vi "stage 2.vi"() -> (0 "pass":bool=TRUE, 1 "Boolean 5":bool, 2 "Boolean 7":bool, 3 "Boolean 8":bool)   [LabVIEW 2014]
uses:
  <vilib>/Utility/miscctls.llb/LVPositionTypeDef.ctl
panel:
  in  "Position 2":T1={"Left"=264, "Top"=264}
  in  "hh":dbl format="%0#2_6g"
  in  ":":dbl format="%0#2_6g"
  in  "ss":dbl format="%0#2_6g"
  out "star 1":bool
  out "star 2":bool
  out "star 3":bool
  out "Boolean 3":bool
  out "Boolean":bool
  out "Boolean 2":bool
  out "Boolean 4":bool
  out "result":bool
  in  "Boolean 6":bool
  in  "Position":T1
  in  "character":bool
  in  "Map Array":dbl[][](array[numeric])=array120x120[14400 elements]
  in  "OK Button 44":bool
  in  "OK Button 43":bool
  in  "OK Button 42":bool
  in  "OK Button 41":bool
  in  "OK Button 40":bool
  in  "OK Button 39":bool
  in  "stop 2":bool
  in  "OK Button 38":bool
  in  "OK Button 37":bool
  in  "OK Button 36":bool
  in  "OK Button 35":bool
  in  "OK Button 34":bool
  in  "OK Button 33":bool
  in  "OK Button 32":bool
  in  "OK Button 29":bool
  in  "OK Button 31":bool
  in  "OK Button 28":bool
  in  "OK Button 27":bool
  in  "OK Button 30":bool
  in  "OK Button 26":bool
  in  "OK Button 25":bool
  in  "OK Button 24":bool
  in  "OK Button 23":bool
  in  "stop":bool
  in  "OK Button 22":bool
  in  "OK Button 21":bool
  in  "OK Button 20":bool
  in  "OK Button 19":bool
  in  "OK Button 18":bool
  in  "OK Button 17":bool
  in  "OK Button 16":bool
  in  "OK Button 15":bool
  in  "OK Button 14":bool
  in  "OK Button 13":bool
  in  "OK Button 12":bool
  in  "OK Button 11":bool
  in  "OK Button 10":bool
  in  "OK Button 9":bool
  in  "OK Button 8":bool
  in  "OK Button 7":bool
  in  "OK Button 6":bool
  in  "OK Button 5":bool
  in  "OK Button 4":bool
  in  "OK Button 3":bool
  in  "OK Button":bool
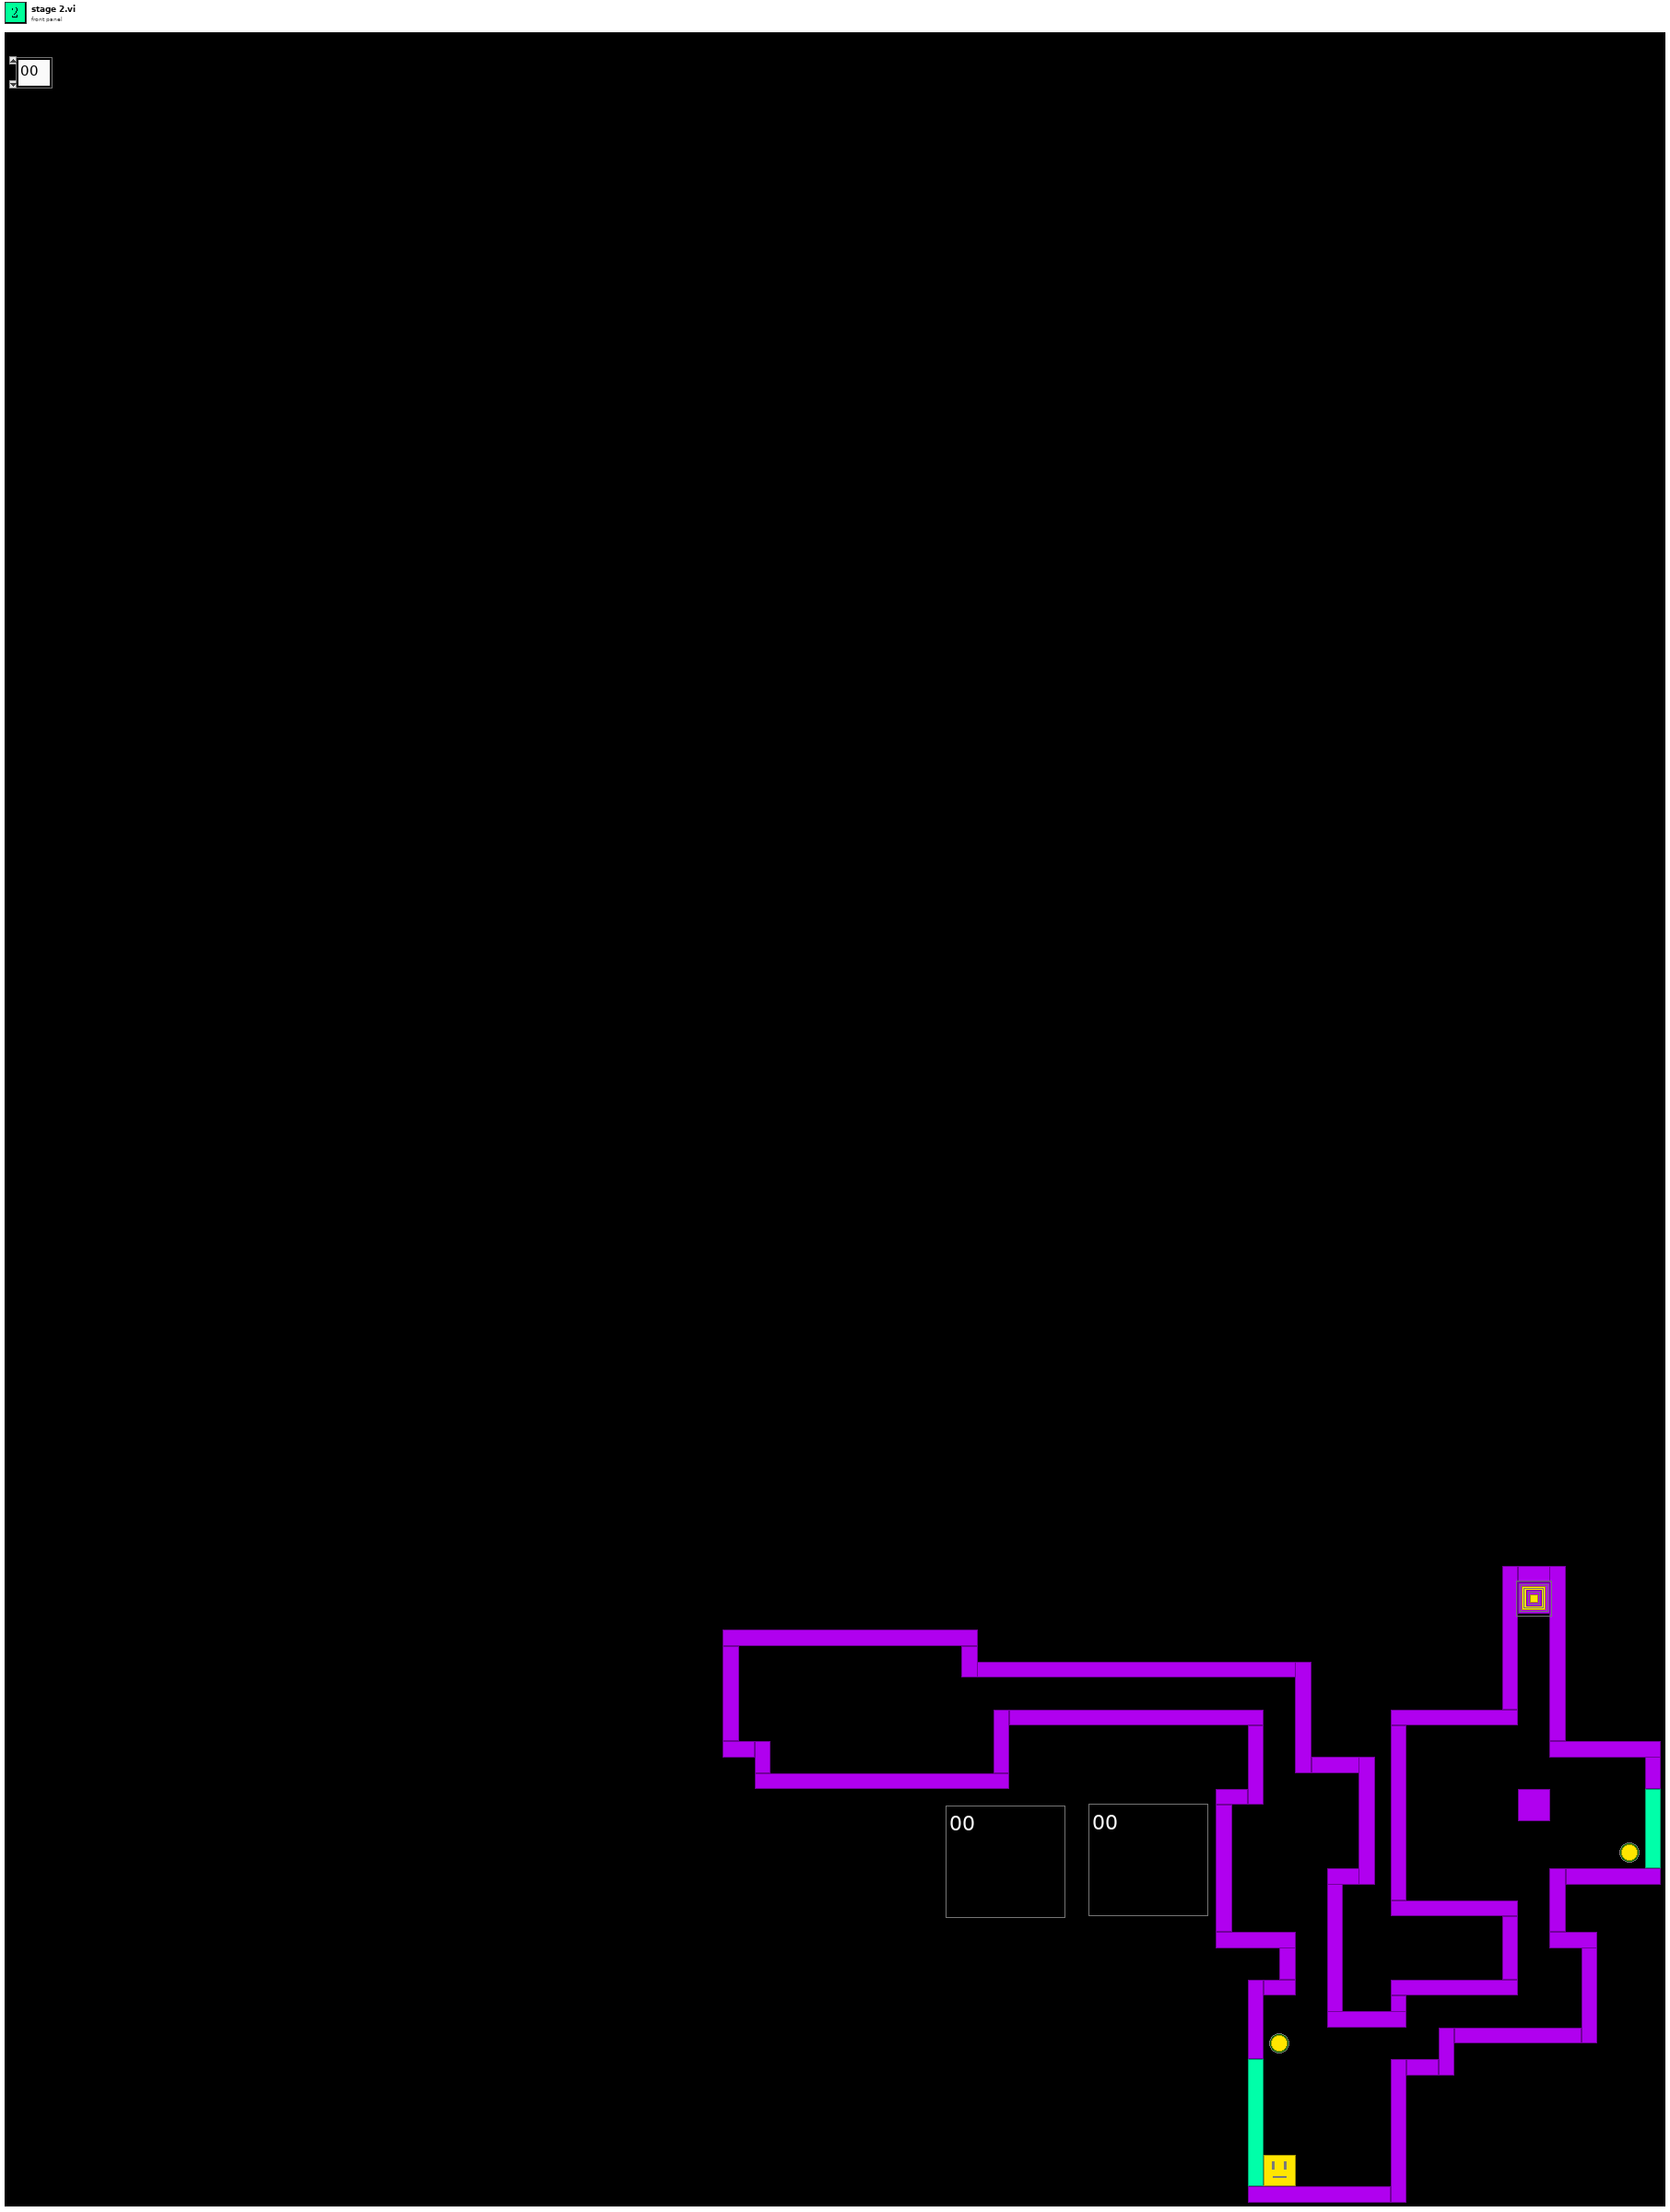
[diagram p1: front panel]
types:
  T1 = typedef "LVPositionTypeDef.ctl" = cluster{"Left":i32, "Top":i32}
  T2 = typedef "eventvkey.ctl" = enum16{"ASCII", "Enter", "Return", "Shift", "Ctrl", "Alt", "Cmd", "Opt", "Caps", "NumLock", "Clear", "Break", "Up", "Down", "Left", "Right", "Insert", "Delete", "Home", "End", "PageUp", "PageDown", "Escape", "Help", "Pause", "ScrollLock", "F1", "F2", "F3", "F4", "F5", "F6", "F7", "F8", "F9", "F10", "F11", "F12", "F13", "F14", "F15", "F16", "F17", "F18", "F19", "F20", "F21", "F22", "F23", "F24", "Play", "VolumeUp", "VolumeDown", "Mute", "Two Byte Char"}
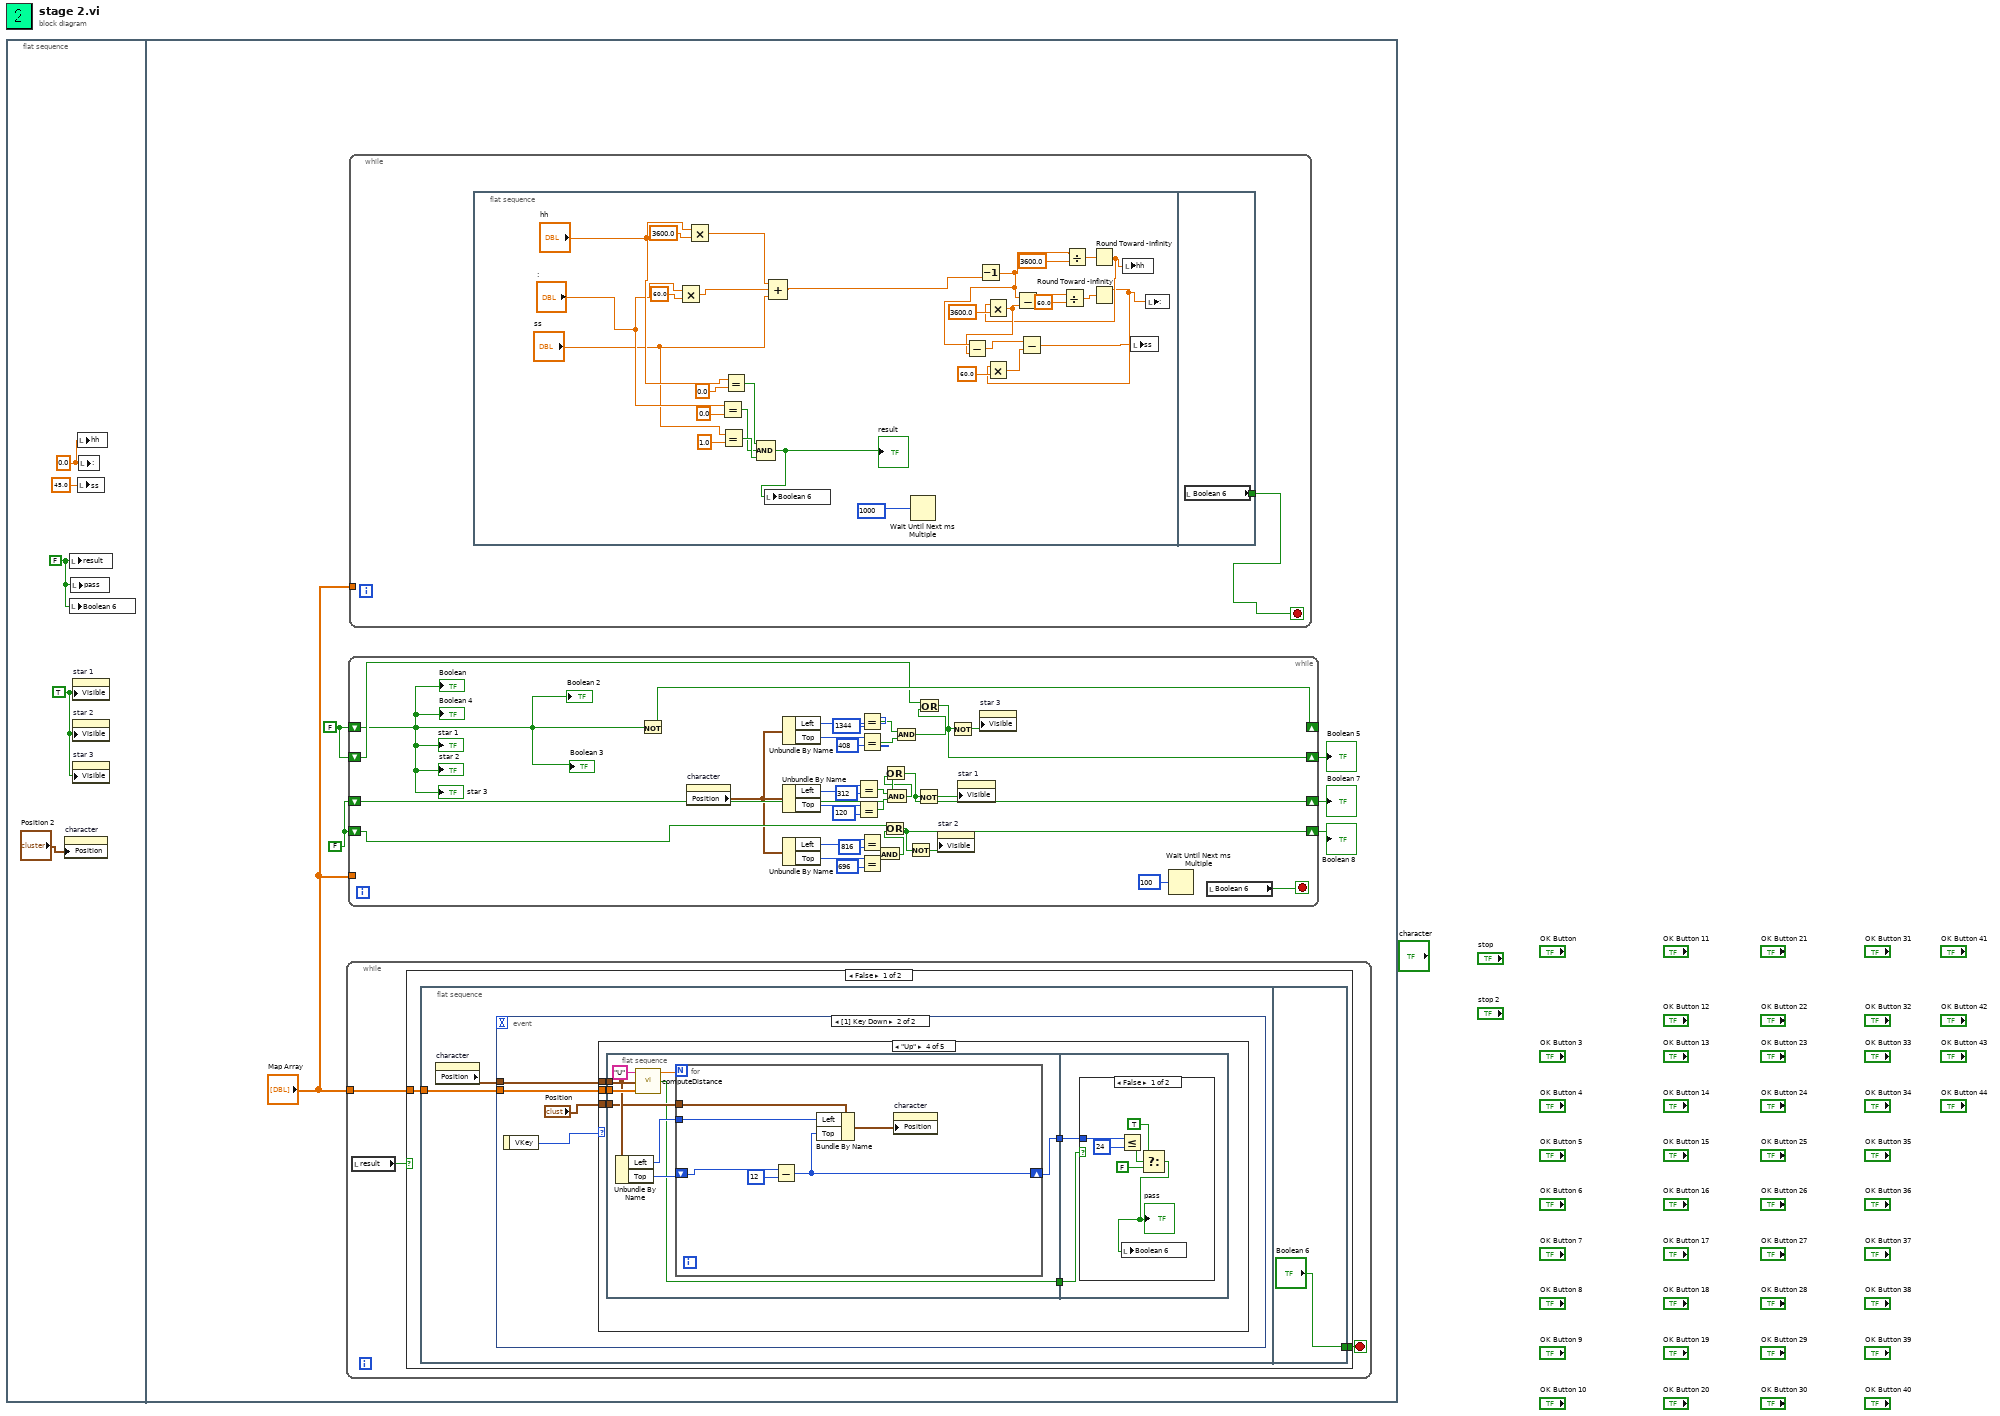
[diagram p0: block diagram]
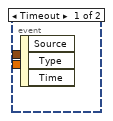
[diagram p2: hidden frame]
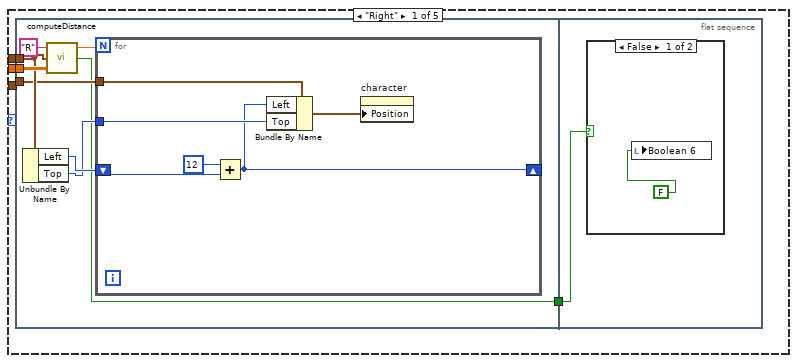
[diagram p3: hidden frame]
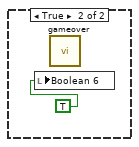
[diagram p4: hidden frame]
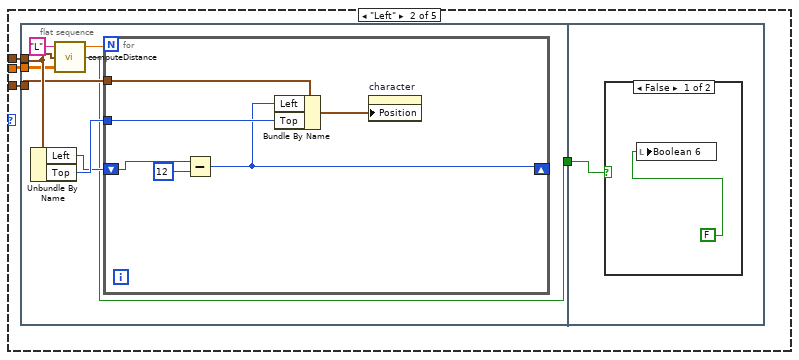
[diagram p5: hidden frame]
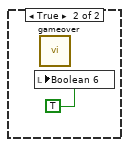
[diagram p6: hidden frame]
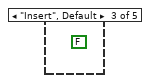
[diagram p7: hidden frame]
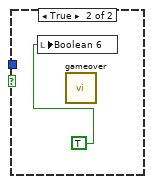
[diagram p8: hidden frame]
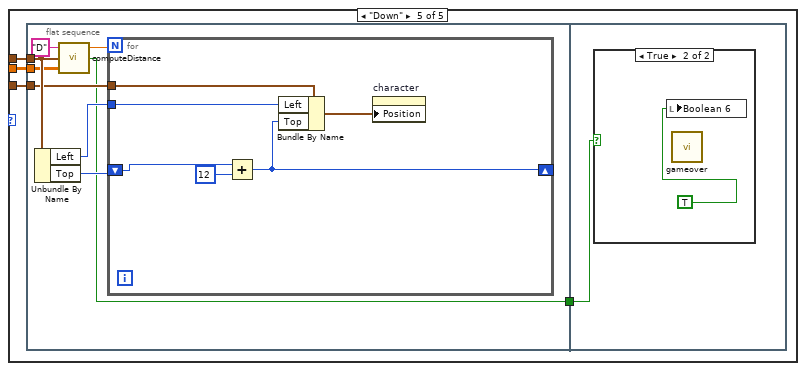
[diagram p9: hidden frame]
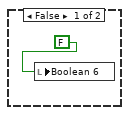
[diagram p10: hidden frame]
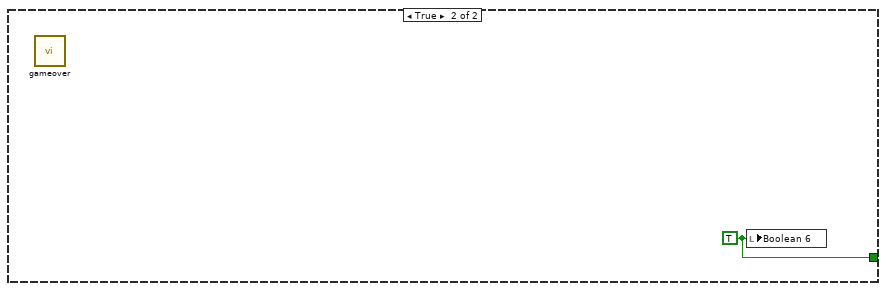
[diagram p11: hidden frame]
diagram:
  n1 = flat-sequence {
    frame #0 {
      w3 = TRUE ("Visible")
      w2 = FALSE ("result")
      w4 = 0.0 (":")
      n2 = property on="character" class="Bool"("Position"="Position 2") -> ()  [unwired: 2 in, 2 out]
      n3 = local write "result"(w2) -> ()
      n4 = local write "Boolean 6"(w2) -> ()
      n5 = local write "pass"(w2) -> ()
      n6 = property on="star 1" class="Bool (strict)"("Visible"=w3) -> ()  [unwired: 2 in, 2 out]
      n7 = property on="star 2" class="Bool (strict)"("Visible"=w3) -> ()  [unwired: 2 in, 2 out]
      n8 = property on="star 3" class="Bool (strict)"("Visible"=w3) -> ()  [unwired: 2 in, 2 out]
      n9 = local write "hh"(w4) -> ()
      n10 = local write "ss"(45.0 ("ss")) -> ()
      n11 = local write ":"(w4) -> ()
    }
    frame #1 {
      w10 = FALSE
      w11 = FALSE
      n12 = while {
        tunnel: "Map Array" -> [w81]
        stop <- w80 stop-if-true
        n13 = local read "result"() -> (w79:bool)
        n14 = case shown="False" w79 {
          tunnel: w81 -> [w83 _]
          tunnel: [w82 w183] -> w80
          frame False {
            n15 = flat-sequence {
              tunnel: w83 -> [w85]
              tunnel: ["Boolean 6"] -> w82
              frame #0 {
                n16 = property on="character" class="Bool"() -> ("Position"=w84:T1)  [unwired: 2 in, 2 out]
                n17 = event shown="[1] Key Down" {
                  selector: _ -> [_ _]
                  dyn-events: _ -> [_ _]
                  timeout: _ -> [_ _]
                  tunnel: w85 -> [_ w88]
                  tunnel: w84 -> [_ w87]
                  event Timeout {
                    n18 = event-data() -> ()  [unwired: 1 in, 3 out]
                  }
                  event Key Down {
                    n19 = event-data() -> ("VKey"=w89:T2)  [unwired: 1 in]
                    n20 = case shown="\"Up\"" w89 {
                      tunnel: w88 -> [w93 w113 _ w136 w163]
                      tunnel: w87 -> [w92 w114 _ w135 w164]
                      tunnel: "Position" -> [w91 w112 _ w134 w162]
                      frame "Right" {
                        n21 = flat-sequence {
                          tunnel: w93 -> [w99]
                          tunnel: w92 -> [w98]
                          tunnel: w91 -> [w97]
                          tunnel: [w94] -> w90
                          tunnel: w90 -> [w108]
                          frame #0 {
                            n22 = Unbundle By Name(w98) -> ("Left"=w96:i32, "Top"=w95:i32)
                            n23 = call "computeDistance.vi"("Array"=w99, "Position"=w98, "String"="R") -> ("2"=w94:bool, "distance"=w101:dbl)  [unwired: 1 out]
                            n24 = for {
                              N: w101 -> [_]
                              shift-right: [w104] -> _
                              shift-left: w96 -> [w107]
                              tunnel: w97 -> [w106]
                              tunnel: w95 -> [w105]
                              n25 = Add(x=12, y=w107) -> (x+y=w104:i32)
                              n26 = Bundle By Name(cluster=w106, "Left"=w104, "Top"=w105) -> (w102:T1)
                              n27 = property on="character" class="Bool"("Position"=w102) -> ()  [unwired: 2 in, 2 out]
                            }
                          }
                          frame #1 {
                            n28 = case shown="False" w108 {
                              frame False {
                                n29 = local write "Boolean 6"(FALSE) -> ()
                              }
                              frame True {
                                n30 = local write "Boolean 6"(TRUE) -> ()
                                n31 = call "gameover.vi"() -> ()  [unwired: 1 in]
                              }
                            }
                          }
                        }
                      }
                      frame "Left" {
                        n32 = flat-sequence {
                          tunnel: w114 -> [w118]
                          tunnel: w113 -> [w117]
                          tunnel: w112 -> [w116]
                          tunnel: [w115] -> w111
                          tunnel: w111 -> [w129]
                          frame #0 {
                            n33 = Unbundle By Name(w118) -> ("Left"=w121:i32, "Top"=w122:i32)
                            n34 = call "computeDistance.vi"("Array"=w117, "Position"=w118, "String"="L") -> ("2"=w115:bool, "distance"=w119:dbl)  [unwired: 1 out]
                            n35 = for {
                              N: w119 -> [_]
                              shift-right: [w126] -> _
                              shift-left: w121 -> [w125]
                              tunnel: w116 -> [w128]
                              tunnel: w122 -> [w127]
                              n36 = Subtract(x=w125, y=12) -> (x-y=w126:i32)
                              n37 = Bundle By Name(cluster=w128, "Left"=w126, "Top"=w127) -> (w123:T1)
                              n38 = property on="character" class="Bool"("Position"=w123) -> ()  [unwired: 2 in, 2 out]
                            }
                          }
                          frame #1 {
                            n39 = case shown="False" w129 {
                              frame False {
                                n40 = local write "Boolean 6"(FALSE) -> ()
                              }
                              frame True {
                                n41 = local write "Boolean 6"(TRUE) -> ()
                                n42 = call "gameover.vi"() -> ()  [unwired: 1 in]
                              }
                            }
                          }
                        }
                      }
                      frame "Insert", Default {
                        (unwired) FALSE
                      }
                      frame "Up" {
                        n43 = flat-sequence {
                          tunnel: w136 -> [w145]
                          tunnel: w135 -> [w142]
                          tunnel: w134 -> [w139]
                          tunnel: [w138] -> w133
                          tunnel: [w137] -> w132
                          tunnel: w133 -> [w153]
                          tunnel: w132 -> [w152]
                          frame #0 {
                            n44 = Unbundle By Name(w142) -> ("Left"=w140:i32, "Top"=w141:i32)
                            n45 = call "computeDistance.vi"("Array"=w145, "Position"=w142, "String"="U") -> ("2"=w138:bool, "distance"=w143:dbl)  [unwired: 1 out]
                            n46 = for {
                              N: w143 -> [_]
                              shift-right: [w151] -> w137
                              shift-left: w141 -> [w148]
                              tunnel: w140 -> [w150]
                              tunnel: w139 -> [w149]
                              n47 = Subtract(x=w148, y=12) -> (x-y=w151:i32)
                              n48 = Bundle By Name(cluster=w149, "Left"=w150, "Top"=w151) -> (w146:T1)
                              n49 = property on="character" class="Bool"("Position"=w146) -> ()  [unwired: 2 in, 2 out]
                            }
                          }
                          frame #1 {
                            n50 = case shown="False" w153 {
                              tunnel: w152 -> [w159 _]
                              frame False {
                                n51 = Less Or Equal?(x=w159, y=24) -> (x <= y?=w157:bool)
                                n52 = Select(t=TRUE, s=w157, f=FALSE) -> (s? t:f=w155:bool)
                                "pass" <- w155
                                n53 = local write "Boolean 6"(w155) -> ()
                              }
                              frame True {
                                n54 = local write "Boolean 6"(TRUE) -> ()
                                n55 = call "gameover.vi"() -> ()  [unwired: 1 in]
                              }
                            }
                          }
                        }
                      }
                      frame "Down" {
                        n56 = flat-sequence {
                          tunnel: w164 -> [w168]
                          tunnel: w163 -> [w167]
                          tunnel: w162 -> [w166]
                          tunnel: [w165] -> w161
                          tunnel: w161 -> [w179]
                          frame #0 {
                            n57 = Unbundle By Name(w168) -> ("Left"=w172:i32, "Top"=w171:i32)
                            n58 = call "computeDistance.vi"("Array"=w167, "Position"=w168, "String"="D") -> ("2"=w165:bool, "distance"=w170:dbl)  [unwired: 1 out]
                            n59 = for {
                              N: w170 -> [_]
                              shift-right: [w178] -> _
                              shift-left: w171 -> [w175]
                              tunnel: w172 -> [w177]
                              tunnel: w166 -> [w176]
                              n60 = Add(x=w175, y=12) -> (x+y=w178:i32)
                              n61 = Bundle By Name(cluster=w176, "Left"=w177, "Top"=w178) -> (w173:T1)
                              n62 = property on="character" class="Bool"("Position"=w173) -> ()  [unwired: 2 in, 2 out]
                            }
                          }
                          frame #1 {
                            n63 = case shown="True" w179 {
                              frame False {
                                n64 = local write "Boolean 6"(FALSE ("Boolean 6")) -> ()
                              }
                              frame True {
                                n65 = local write "Boolean 6"(TRUE) -> ()
                                n66 = call "gameover.vi"() -> ()  [unwired: 1 in]
                              }
                            }
                          }
                        }
                      }
                    }
                  }
                }
              }
              frame #1 {
              }
            }
          }
          frame True {
            w183 = TRUE ("Boolean 6")
            n67 = call "gameover.vi"() -> ()  [unwired: 1 in]
            n68 = local write "Boolean 6"(w183) -> ()
          }
        }
      }
      n69 = while {
        shift-right: [w77] -> _
        shift-left: w11 -> [w44]
        shift-right: [w66] -> w7
        shift-left: w10 -> [w68]
        shift-right: [w57] -> w6
        shift-left: w10 -> [w56]
        shift-right: [w46] -> w8
        shift-left: w11 -> [w45]
        tunnel: "Map Array" -> [_]
        stop <- w76 stop-if-true
        n70 = Not(x=w44) -> (.not. x?=w77:bool)
        n71 = property on="character" class="Bool"() -> ("Position"=w47:T1)  [unwired: 2 in, 2 out]
        n72 = Unbundle By Name(w47) -> ("Left"=w55:i32, "Top"=w53:i32)
        n73 = Unbundle By Name(w47) -> ("Left"=w75:i32, "Top"=w73:i32)
        n74 = Unbundle By Name(w47) -> ("Left"=w58:i32, "Top"=w60:i32)
        n75 = Equal?(x=w75, y=312) -> (x = y?=w71:bool)
        n76 = Equal?(x=w73, y=120) -> (x = y?=w70:bool)
        n77 = Equal?(x=w55, y=1344) -> (x = y?=w51:bool)
        n78 = Equal?(x=w53, y=408) -> (x = y?=w50:bool)
        n79 = Equal?(x=w58, y=816) -> (x = y?=w62:bool)
        n80 = Equal?(x=w60, y=696) -> (x = y?=w63:bool)
        n81 = And(x=w62, y=w63) -> (x .and. y?=w65:bool)
        n82 = Or(x=w56, y=w65) -> (x .or. y?=w57:bool)
        n83 = And(x=w71, y=w70) -> (x .and. y?=w67:bool)
        n84 = Or(x=w68, y=w67) -> (x .or. y?=w66:bool)
        n85 = And(x=w51, y=w50) -> (x .and. y?=w48:bool)
        n86 = Not(x=w57) -> (.not. x?=w64:bool)
        n87 = Not(x=w66) -> (.not. x?=w69:bool)
        n88 = Or(x=w45, y=w48) -> (x .or. y?=w46:bool)
        n89 = property on="star 2" class="Bool (strict)"("Visible"=w64) -> ()  [unwired: 2 in, 2 out]
        n90 = Not(x=w46) -> (.not. x?=w49:bool)
        n91 = property on="star 1" class="Bool (strict)"("Visible"=w69) -> ()  [unwired: 2 in, 2 out]
        n92 = property on="star 3" class="Bool (strict)"("Visible"=w49) -> ()  [unwired: 2 in, 2 out]
        n93 = Wait Until Next ms Multiple(millisecond multiple=u32 100) -> ()  [unwired: 1 out]
        n94 = local read "Boolean 6"() -> (w76:bool)
        "star 1" <- w44
        "star 2" <- w44
        "star 3" <- w44
        "Boolean" <- w44
        "Boolean 4" <- w44
        "Boolean 2" <- w44
        "Boolean 3" <- w44
      }
      "Boolean 5" <- w8
      "Boolean 7" <- w7
      "Boolean 8" <- w6
      n95 = while {
        tunnel: "Map Array" -> [_]
        stop <- w12 stop-if-true
        n96 = flat-sequence {
          tunnel: [w43] -> w12
          frame #0 {
            n97 = Multiply(x=":", y=60.0) -> (x*y=w41:dbl)
            n98 = Multiply(x="hh", y=3600.0) -> (x*y=w42:dbl)
            n99 = Equal?(x=":", y=0.0) -> (x = y?=w33:bool)
            n100 = Equal?(x="ss", y=1.0) -> (x = y?=w34:bool)
            n101 = Equal?(x="hh", y=0.0) -> (x = y?=w32:bool)
            n102 = Compound Arithmetic op=AND(w32, w33, w34) -> (w13:bool)
            "result" <- w13
            n103 = local write "Boolean 6"(w13) -> ()
            n104 = Compound Arithmetic op=ADD(w42, w41, "ss") -> (w38:dbl)
            n105 = Wait Until Next ms Multiple(millisecond multiple=u32 1000) -> ()  [unwired: 1 out]
            n106 = Decrement(x=w38) -> (x-1=w27:dbl)
            n107 = Divide(x=w27, y=3600.0) -> (x/y=w17:dbl)
            n108 = Round Toward -Infinity(1:w17) -> (0:w16:dbl)
            n109 = Multiply(x=w16, y=3600.0) -> (x*y=w23:dbl)
            n110 = Subtract(x=w27, y=w23) -> (x-y=w24:dbl)
            n111 = Subtract(x=w27, y=w23) -> (x-y=w20:dbl)
            n112 = Divide(x=w20, y=60.0) -> (x/y=w22:dbl)
            n113 = Round Toward -Infinity(1:w22) -> (0:w15:dbl)
            n114 = Multiply(x=w15, y=60.0) -> (x*y=w26:dbl)
            n115 = Subtract(x=w24, y=w26) -> (x-y=w14:dbl)
            n116 = local write "hh"(w16) -> ()
            n117 = local write "ss"(w14) -> ()
            n118 = local write ":"(w15) -> ()
          }
          frame #1 {
            n119 = local read "Boolean 6"() -> (w43:bool)
          }
        }
      }
    }
  }
